vi "nonreentrant out.vi"(8 "error in (no error)":errorcluster, 10 "data table in":T1, 11 "Queue in":refnum<queue>) -> (0 "error out":errorcluster)   [LabVIEW 2013, in "testmod runtime.lvclass"]
uses:
  testmod runtime.lvclass
  <vilib>/NI/Tag Bus/table/data table.ctl
  <vilib>/NI/Tag Bus/table/data table.lvlib
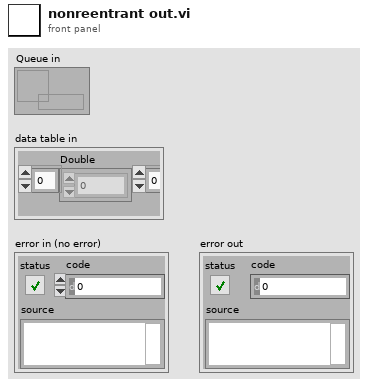
[diagram p1: front panel]
types:
  T1 = typedef "tag bus.lvlib/data table.lvlib/data table.ctl" = cluster{"Double":dbl[], "Single":sgl[], "I64":i64[], "I32":i32[], "I16":i16[], "I8":i8[], "U64":u64[], "U32":u32[], "U16":u16[], "U8":u8[], "Boolean":bool[], "String":string[], "Array of Double":cluster{"DBL Array":dbl[]}[], "Array of Single":cluster{"SGL Array":sgl[]}[], "Array of I64":cluster{"I64 Array":i64[]}[], "Array of I32":cluster{"I32 Array":i32[]}[], "Array of I16":cluster{"I16 Array":i16[]}[], "Array of I8":cluster{"I8 Array":i8[]}[], "Array of U64":cluster{"U64 Array":u64[]}[], "Array of U32":cluster{"U32 Array":u32[]}[], "Array of U16":cluster{"U16 Array":u16[]}[], "Array of U8":cluster{"U8 Array":u8[]}[], "Array of Boolean":cluster{"Boolean Array":bool[]}[], "Array of String":cluster{"String Array":string[]}[]}
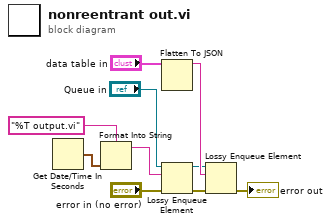
[diagram p0: block diagram]
diagram:
  n1 = Get Date/Time In Seconds() -> (seconds since 1Jan1904=w2:timestamp)
  n2 = Format Into String(format string="%T output.vi", w2) -> (resulting string=w1:string)  [unwired: 2 in, 1 out]
  n3 = Flatten To JSON(anything="data table in") -> (JSON string=w10:string)  [unwired: 2 in, 1 out]
  n4 = Lossy Enqueue Element(queue="Queue in", element=w1, error in (no error)="error in (no error)") -> (queue out=w8:refnum<queue>, error out=w6:errorcluster)  [unwired: 2 out]
  n5 = Lossy Enqueue Element(queue=w8, element=w10, error in (no error)=w6) -> (error out=→"error out":errorcluster)  [unwired: 3 out]
